vi "Write to File.vi"(8 "error in (no error)":errorcluster, 9 "Flush After Write?":bool, 10 "Data to Write":string, 11 "Text File in":refnum<class "Text File.lvclass">) -> (0 "error out":errorcluster, 3 "Text File out":refnum<class "Text File.lvclass">)   [LabVIEW 2020, in "Text File.lvclass"]
uses:
  <vilib>/gpm_packages/@cs/event-logger/Source/Text File Sink/Text File/Text File.lvclass
  <vilib>/gpm_packages/@cs/event-logger/Source/Text File Sink/Text File/Text File.lvclass/Text File.ctl
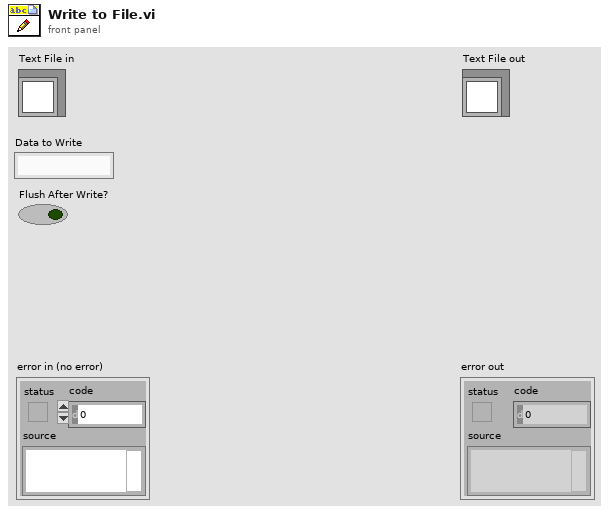
[diagram p1: front panel]
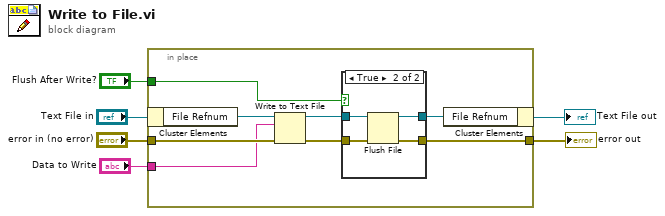
[diagram p0: block diagram]
diagram:
  n1 = in-place {
    in-place-border: "error in (no error)" -> [w13]
    in-place-border: [w8] -> w3
    in-place-border: "Data to Write" -> [w12]
    in-place-border: "Flush After Write?" -> [w7]
    n2 = in-place-cluster #1("Text File in") -> ("File Refnum"=w14:refnum<file>)
    n3 = Write to Text File(file (use dialog)=w14, text=w12, error in=w13) -> (refnum out=w11:refnum<file>, error out=w10:errorcluster)  [unwired: 1 in, 1 out]
    n4 = case shown="True" w7 {
      tunnel: w11 -> [w16 w20]
      tunnel: w10 -> [w15 w19]
      tunnel: [w16 w18] -> w9
      tunnel: [w15 w17] -> w8
      frame False {
      }
      frame True {
        n5 = Flush File(refnum=w20, error in=w19) -> (refnum out=w18:refnum<file>, error out=w17:errorcluster)
      }
    }
    n6 = in-place-cluster #1("File Refnum"=w9) -> (→"Text File out":refnum<class "Text File.lvclass">)
  }
  "error out" <- w3
